vi "Day 11 - Part two.vi"() -> ()   [LabVIEW 2023]
uses:
  <vilib>/Utility/error.llb/Trim Whitespace One-Sided.vi
panel:
  out "i":i32
  out "Array":u64[][][](array[numeric])
  out "inspected items":u64[](array[numeric])
  out "Monkeys":T1(array[cluster])
  out "Answer 2":u64
  in  "test":bool
  in  "test input":string="Monkey 0:\n  Starting items: 79, 98\n  Operation: new = old * 19\n  Test: divisible by 23\n    If true: throw to monkey 2\n    If false: throw to monkey 3\n\nMonkey 1:\n  Starting items: 54, 65, 75, 74\n  Operation: new = old + 6\n  Test: divisible by 19\n    If true: throw to monkey 2\n    If false: throw to monkey 0\n\nMonkey 2:\n  Starting items: 79, 60, 97\n  Operation: new = old * old\n  Test: divisible by 13\n    If true: throw to monkey 1\n    If false: throw to monkey 3\n\nMonkey 3:\n  Starting items: 74\n  Operation: new = old + 3\n  Test: divisible by 17\n    If true: throw to monkey 0\n    If false: throw to monkey 1"
  in  "input":string="Monkey 0:\n  Starting items: 57, 58\n  Operation: new = old * 19\n  Test: divisible by 7\n    If true: throw to monkey 2\n    If false: throw to monkey 3\n\nMonkey 1:\n  Starting items: 66, 52, 59, 79, 94, 73\n  Operation: new = old + 1\n  Test: divisible by 19\n    If true: throw to monkey 4\n    If false: throw to monkey 6\n\nMonkey 2:\n  Starting items: 80\n  Operation: new = old + 6\n  Test: divisible by 5\n    If true: throw to monkey 7\n    If false: throw to monkey 5\n\nMonkey 3:\n  Starting items: 82, 81, 68, 66, 71, 83, 75, 97\n  Operation: new = old + 5\n  Test: divisible by 11\n    If true: throw to monkey 5\n    If false: throw to monkey 2\n\nMonkey 4:\n  Starting items: 55, 52, 67, 70, 69, 94, 90\n  Operation: new = old * old\n  Test: divisible by 17\n    If true: throw to monkey 0\n    If false: throw to monkey 3\n\nMonkey 5:\n  Starting items: 69, 85, 89, 91\n  Operation: new = old + 7\n  Test: divisible by 13\n    If true: throw to monkey 1\n    If false: throw to monkey 7\n\nMonkey 6:\n  Starting items: 75, 53, 73, 52, 75\n  Operation: new = old * 7\n  Test: divisible by 2\n    If true: throw to monkey 0\n    If false: throw to monkey 4\n\nMonkey 7:\n  Starting items: 94, 60, 79\n  Operation: new = old + 2\n  Test: divisible by 3\n    If true: throw to monkey 1\n    If false: throw to monkey 6\n"
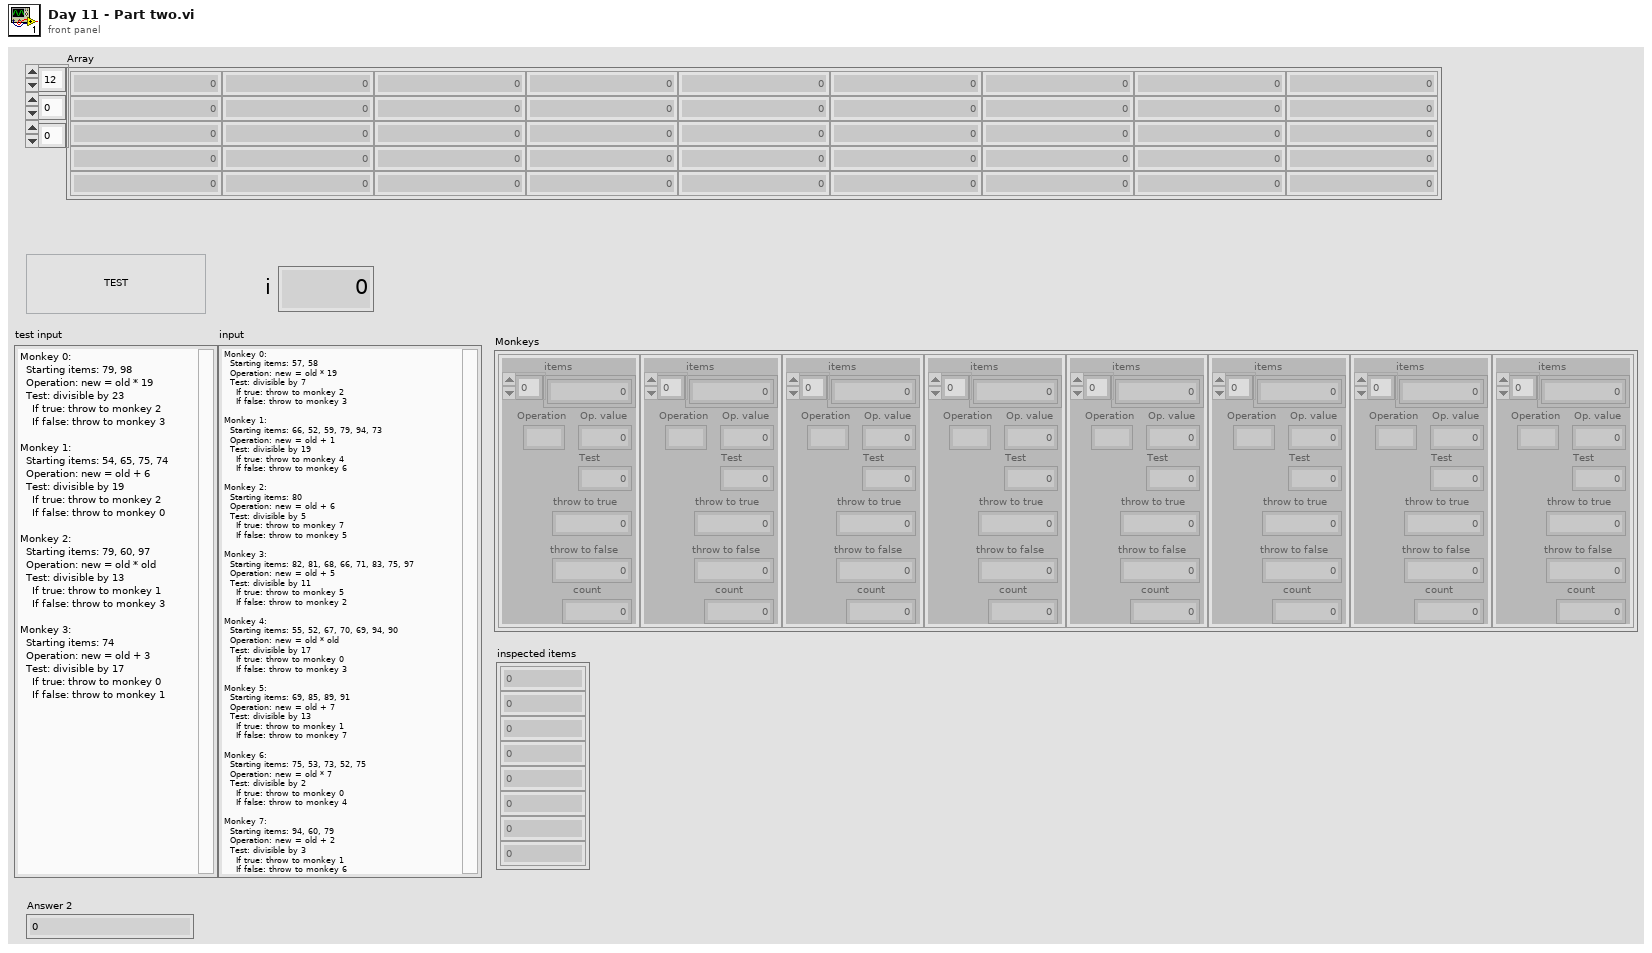
[diagram p1: front panel]
types:
  T1 = cluster{"items":u64[], "Operation":string, "Op. value":i32, "throw to true":i32, "throw to false":i32, "Test":i32, "count":u64}[]
  T2 = cluster{"items":u64[], "Operation":string, "Op. value":i32, "throw to true":i32, "throw to false":i32, "Test":i32, "count":u64}
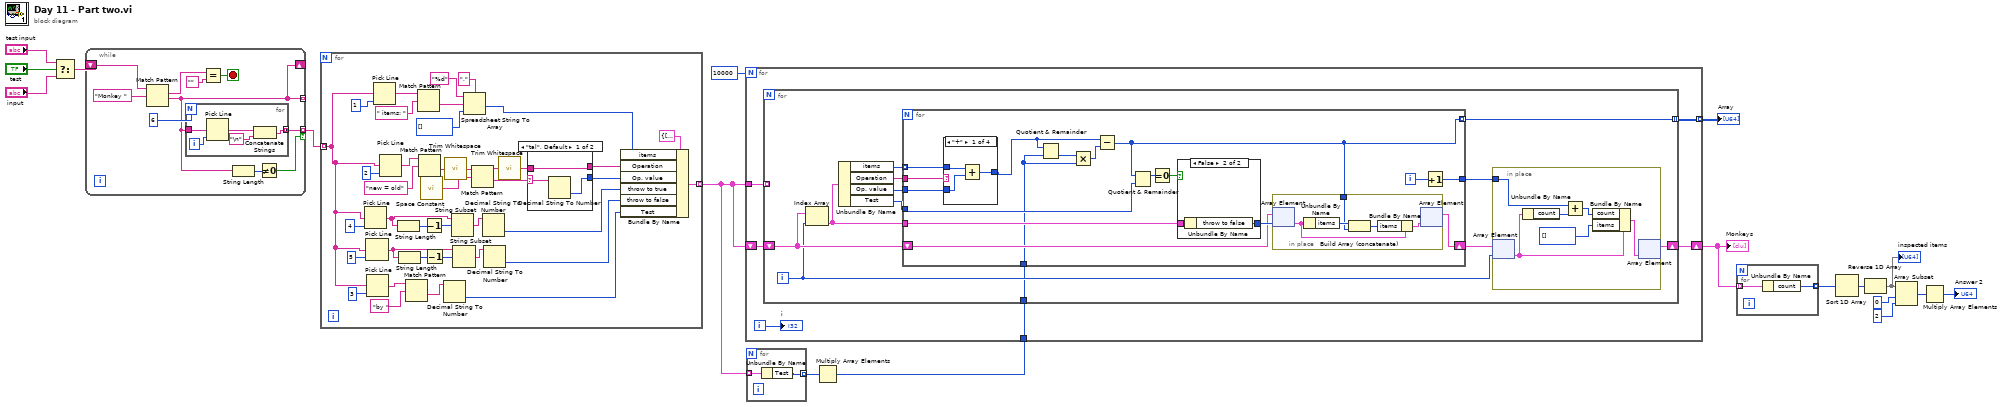
[diagram p0: block diagram]
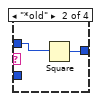
[diagram p2: hidden frame]
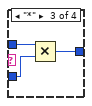
[diagram p3: hidden frame]
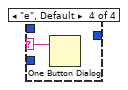
[diagram p4: hidden frame]
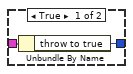
[diagram p5: hidden frame]
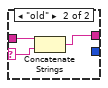
[diagram p6: hidden frame]
diagram:
  n1 = Select(t="test input", s="test", f="input") -> (s? t:f=w14:string)
  n2 = while {
    shift-right: [w19] -> _
    shift-left: w14 -> [w28]
    tunnel: [w21] -> w15 mode=indexing if=w20
    tunnel: [w19] -> _ mode=indexing
    stop <- w23 stop-if-true
    n3 = Match Pattern(string=w28, regular expression="Monkey ") -> (match substring=w24:string, after substring=w19:string)  [unwired: 1 in, 2 out]
    n4 = for {
      N: 6 -> [_]
      tunnel: w19 -> [w33]
      tunnel: [w30] -> w21 mode=concatenating
      i -> [w31]
      n5 = Pick Line(multi-line string=w33, line index=w31) -> (output string=w32:string)  [unwired: 1 in]
      n6 = Concatenate Strings(w32, "\n") -> (w30:string)
    }
    n7 = Equal?(x=w24, y="") -> (x = y?=w23:bool)
    n8 = String Length(string=w19) -> (length=w22:i32)
    n9 = Not Equal To 0?(x=w22) -> (x != 0?=w20:bool)
  }
  n10 = for {
    tunnel: w15 -> [w38] mode=indexing
    tunnel: [w64] -> w3 mode=indexing
    n11 = Pick Line(multi-line string=w38, line index=4) -> (output string=w47:string)  [unwired: 1 in]
    n12 = Pick Line(multi-line string=w38, line index=5) -> (output string=w49:string)  [unwired: 1 in]
    n13 = Pick Line(multi-line string=w38, line index=3) -> (output string=w42:string)  [unwired: 1 in]
    n14 = Pick Line(multi-line string=w38, line index=1) -> (output string=w70:string)  [unwired: 1 in]
    n15 = Pick Line(multi-line string=w38, line index=2) -> (output string=w62:string)  [unwired: 1 in]
    n16 = String Length(string=w47) -> (length=w54:i32)
    n17 = String Length(string=w49) -> (length=w50:i32)
    n18 = Match Pattern(string=w42, regular expression="by ") -> (after substring=w41:string)  [unwired: 1 in, 3 out]
    n19 = Match Pattern(string=w70, regular expression=" items: ") -> (after substring=w68:string)  [unwired: 1 in, 3 out]
    n20 = Match Pattern(string=w62, regular expression="new = old") -> (after substring=w60:string)  [unwired: 1 in, 3 out]
    n21 = call <vilib>:"Space Constant.vi"() -> ("String"=w59:string)
    n22 = Decrement(x=w54) -> (x-1=w45:i32)
    n23 = Decrement(x=w50) -> (x-1=w44:i32)
    n24 = Decimal String To Number(string=w41) -> (number=w40:i32)  [unwired: 2 in, 1 out]
    n25 = call <vilib>:"Trim Whitespace.vi"("string"=w60) -> ("trimmed string"=w58:string)  [unwired: 1 in]
    n26 = String Subset(string=w47, offset (0)=w45) -> (substring=w53:string)  [unwired: 1 in]
    n27 = String Subset(string=w49, offset (0)=w44) -> (substring=w51:string)  [unwired: 1 in]
    n28 = Spreadsheet String To Array(delimiter (Tab)="," ("format string"), format string="%d", spreadsheet string=w68, array type (2D Dbl)=i32[] [] ("output array")) -> (array=w65:i32[])
    n29 = Match Pattern(string=w58, regular expression=w59) -> (before substring=w57:string, after substring=w37:string)  [unwired: 1 in, 2 out]
    n30 = Decimal String To Number(string=w53) -> (number=w52:i32)  [unwired: 2 in, 1 out]
    n31 = Decimal String To Number(string=w51) -> (number=w46:i32)  [unwired: 2 in, 1 out]
    n32 = call <vilib>:"Trim Whitespace.vi"("string"=w57) -> ("trimmed string"=w36:string)  [unwired: 1 in]
    n33 = case shown="\"tal\", Default" w37 {
      selector: w37 -> [w74 w77]
      tunnel: [w75 _] -> w56
      tunnel: w36 -> [w73 w78]
      tunnel: [w73 w76] -> w35
      frame "tal", Default {
        n34 = Decimal String To Number(string=w74) -> (number=w75:i32)  [unwired: 2 in, 1 out]
      }
      frame "old" {
        n35 = Concatenate Strings(w78, w77) -> (w76:string)
      }
    }
    n36 = Bundle By Name(cluster=T2 {"items"=[], "Operation"="", "Op. value"=0, "throw to true"=0, "throw to false"=0, "Test"=0, "count"=0} ("input cluster"), "items"=w65, "Operation"=w35, "Op. value"=w56, "throw to true"=w52, "throw to false"=w46, "Test"=w40) -> (w64:T2)
  }
  n37 = for {
    tunnel: w3 -> [w80] mode=indexing
    tunnel: [w79] -> w2 mode=indexing
    n38 = Unbundle By Name(w80) -> ("Test"=w79:i32)
  }
  n39 = Multiply Array Elements(1:w2) -> (0:w1:i32)
  n40 = for {
    N: 10000 -> [_]
    tunnel: w3 -> [w86]
    shift-right: [w85] -> w12
    shift-left: w3 -> [w84]
    tunnel: [w83] -> w4 mode=indexing
    tunnel: w1 -> [w82]
    i -> [w81]
    n41 = for {
      tunnel: w86 -> [_] mode=indexing
      shift-right: [w91] -> w85
      shift-left: w84 -> [w93]
      tunnel: [w88] -> w83 mode=indexing
      tunnel: w82 -> [w87]
      i -> [w89]
      n42 = Index Array(array=w93, index=w89) -> (element=w94:T2)
      n43 = Unbundle By Name(w94) -> ("items"=w98:u64[], "Operation"=w97:string, "Op. value"=w96:i32, "Test"=w95:i32)
      n44 = for {
        tunnel: w98 -> [w114] mode=indexing
        tunnel: w97 -> [w115]
        tunnel: w96 -> [w113]
        tunnel: w95 -> [w112]
        tunnel: w94 -> [w109]
        shift-right: [w107] -> w92
        shift-left: w93 -> [w106]
        tunnel: [w104] -> w90
        tunnel: [w101] -> w88 mode=indexing
        tunnel: w87 -> [w102]
        i -> [w105]
        n45 = case shown="\"+\"" w115 {
          selector: w115 -> [_ _ _ w124]
          tunnel: w114 -> [w117 w119 w123 _]
          tunnel: w113 -> [w116 _ w122 _]
          tunnel: [w118 w120 w121 _] -> w103
          frame "+" {
            n46 = Add(x=w117, y=w116) -> (x+y=w118:u64)
          }
          frame "*old" {
            n47 = Square(x=w119) -> (x^2=w120:u64)
          }
          frame "*" {
            n48 = Multiply(x=w123, y=w122) -> (x*y=w121:u64)
          }
          frame "e", Default {
            n49 = One Button Dialog(message=w124) -> ()  [unwired: 1 in, 1 out]
          }
        }
        n50 = Quotient & Remainder(x=w103, y=w102) -> (floor(x/y)=w100:u64)  [unwired: 1 out]
        n51 = Multiply(x=w100, y=w102) -> (x*y=w99:u64)
        n52 = Subtract(x=w103, y=w99) -> (x-y=w101:u64)
        n53 = Quotient & Remainder(x=w101, y=w112) -> (x-y*floor(x/y)=w111:u64)  [unwired: 1 out]
        n54 = Equal To 0?(x=w111) -> (x = 0?=w110:bool)
        n55 = case shown="False" w110 {
          tunnel: w109 -> [w131 w133]
          tunnel: [w130 w132] -> w108
          frame True {
            n56 = Unbundle By Name(w131) -> ("throw to true"=w130:i32)
          }
          frame False {
            n57 = Unbundle By Name(w133) -> ("throw to false"=w132:i32)
          }
        }
        n58 = in-place {
          in-place-border: w101 -> [w127]
          n59 = in-place-array #1(w106, w108) -> (w125:T2)
          n60 = Unbundle By Name(w125) -> ("items"=w128:u64[])
          n61 = Build Array (concatenate)(w128, w127) -> (w129:u64[])
          n62 = Bundle By Name(cluster=w125, "items"=w129) -> (w126:T2)
          n63 = in-place-array #1(w126) -> (w107:T1)  [unwired: 1 out]
        }
        n64 = Increment(x=w105) -> (x+1=w104:i32)
      }
      n65 = in-place {
        in-place-border: w90 -> [w135]
        n66 = in-place-array #2(w92, w89) -> (w138:T2)
        n67 = Unbundle By Name(w138) -> ("count"=w137:u64)
        n68 = Add(x=w135, y=w137) -> (x+y=w136:u64)
        n69 = Bundle By Name(cluster=w138, "count"=w136, "items"=u64[] []) -> (w139:T2)
        n70 = in-place-array #2(w139) -> (w91:T1)  [unwired: 1 out]
      }
    }
    "i" <- w81
  }
  "Monkeys" <- w12
  "Array" <- w4
  n71 = for {
    tunnel: w12 -> [w141] mode=indexing
    tunnel: [w140] -> w11 mode=indexing
    n72 = Unbundle By Name(w141) -> ("count"=w140:u64)
  }
  n73 = Sort 1D Array(array=w11) -> (sorted array=w10:u64[])
  n74 = Reverse 1D Array(array=w10) -> (reversed array=w5:u64[])
  "inspected items" <- w5
  n75 = Array Subset(array=w5, index=0, length=2) -> (w7:u64[])
  n76 = Multiply Array Elements(1:w7) -> (0:→"Answer 2":u64)
